vi "FTW-Actor.vi"(0 "FTW-TestExecutive-Core":refnum<class "FTW-TestExecutive-Core.lvclass">, 5 "FTW Actor Instance Configuration":string="{\n  \"Identity\": \"FTW Test Executive\",\n  \"InboxAddress\": \"inproc://ftwTestExec\",\n  \"LoggerAddress\": \"\",\n  \"Connections\": {},\n  \"Publishers\": {},\n  \"Subscriptions\": {},\n  \"Step Name Dictionary\": {},\n  \"Refresh Period\": 0.1\n}", 11 "ErrorIn":errorcluster) -> (15 "Error":errorcluster)   [LabVIEW 2015, in "FTW-TestExecutive-Core.lvclass"]
uses:
  FTW-TestExecutive-Core.lvclass
  FTW-TestExecutive-Results.ctl
  FTW-TestExecutive-Core.lvclass/FTW-TestExecutive-Core.ctl
  FTW-TestExecutive-Core_State.ctl
  FTW-TestExecutive-Step-State.ctl
  source/actor/Instance/FTW-ActorInstance.lvclass/FTW-ActorInstance.ctl
  source/JSON/core/FTW-JSON-Core-EncodingFlags.vi
  source/JSON/FTW-JSON-Parse.vi
  source/Reflection/FTW-Reflection-Type.vi
  source/CodeGen/JSON Deserialize/FTW-JSON-Core-GetFlattenedValue.vi
  source/actor/JobSequencer/FTW-SEQ-Current.vi
  source/CodeGen/JSON Deserialize/FTW-JSON-Deserialize.xnode
  source/actor/Message/Base/FTW-Message.lvclass
  source/actor/Connector/FTW-ActorConnector.lvclass
  source/actor/Instance/FTW-ActorInstance.lvclass
  source/actor/Message/Request/FTW-Message-IncomingRequest.lvclass
  source/actor/Instance-Extended/FTW-ActorExtended.lvclass
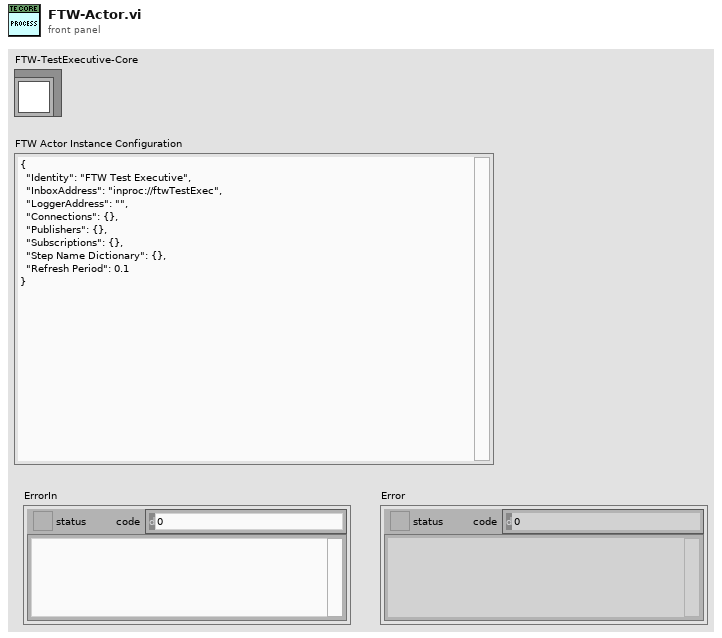
[diagram p1: front panel]
types:
  T1 = cluster{"Incoming Requests":refnum<event-registration>, "Local Messages":refnum<event-registration>, "Subscriber Registration":refnum<event-registration>}
  T2 = typedef "FTW-TestExecutive-Results.ctl" = cluster{"Start Time":timestamp, "Elapsed Time":dbl, "Passed":bool}
  T3 = typedef "FTW-TestExecutive-Step-State.ctl" = enum8{"None", "Failed", "Passed", "Timed out", "Aborted"}
  T4 = typedef "FTW-TestExecutive-Core.lvclass/FTW-TestExecutive-Core_State.ctl" = enum8{"Unloaded", "Loaded", "Executing", "Paused"}
  T5 = typedef "FTW-TestExecutive-Step.ctl" = cluster{"Name":string, "Type":string, "Config":string, "Elapsed Time":dbl, "Passed":bool, "State":T3, "Results":T2}
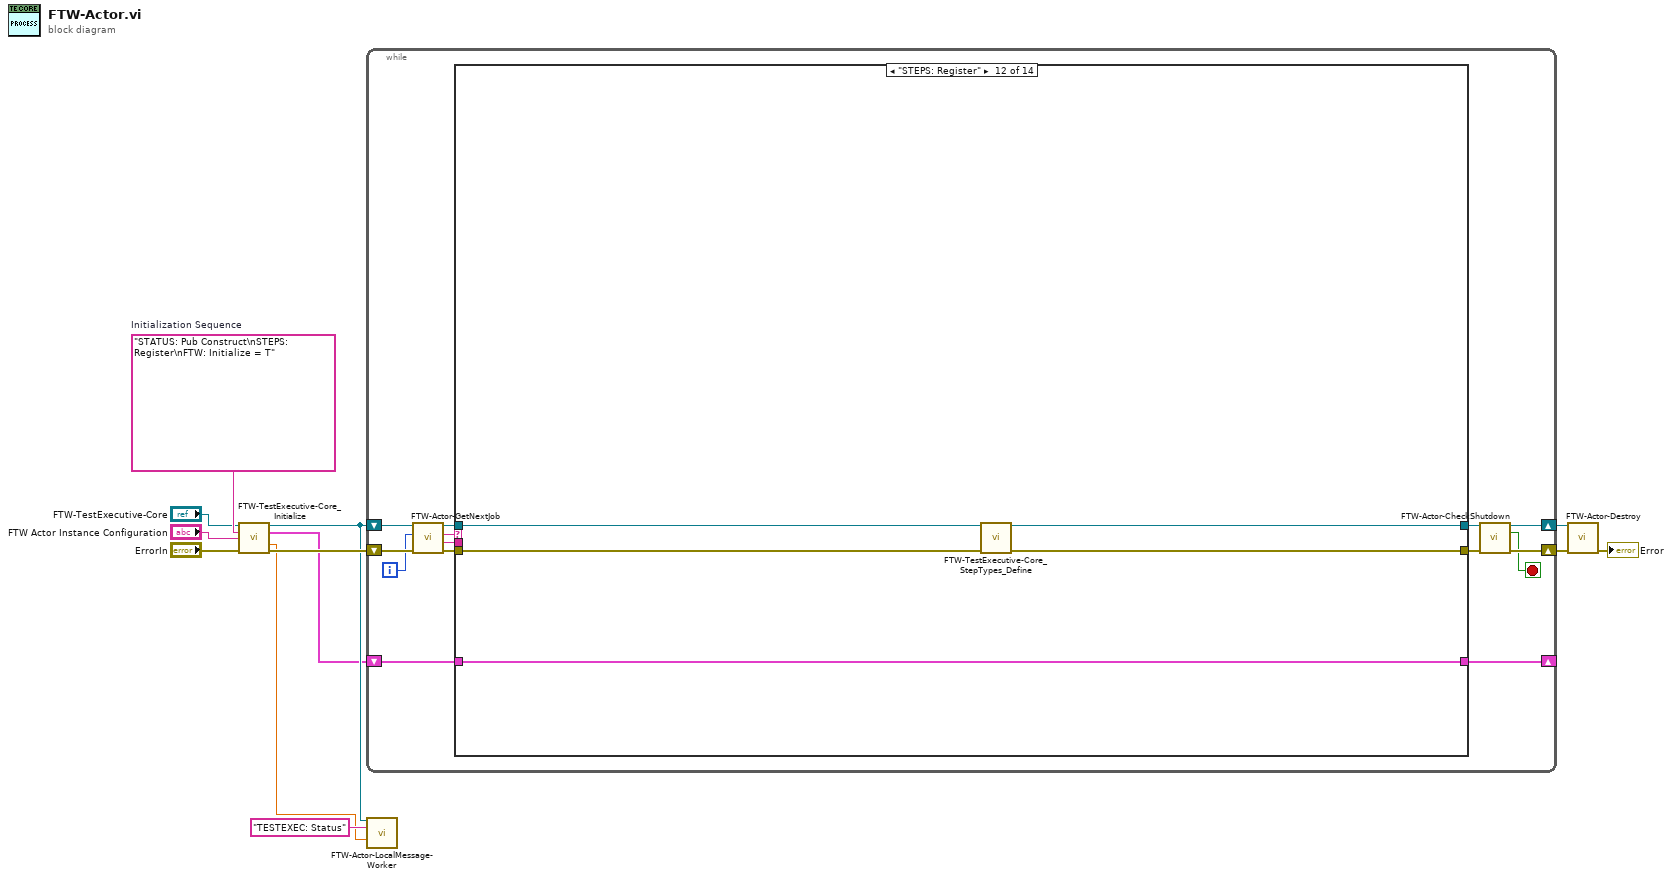
[diagram p0: block diagram]
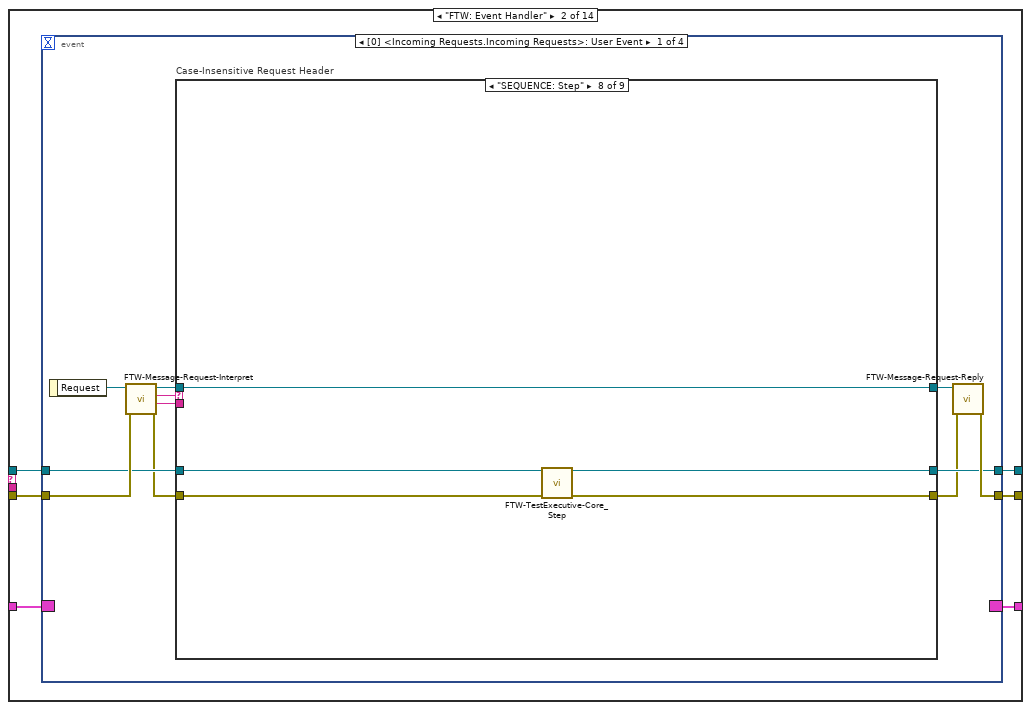
[diagram p3: hidden frame]
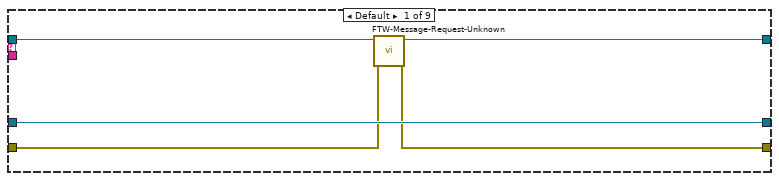
[diagram p4: hidden frame]
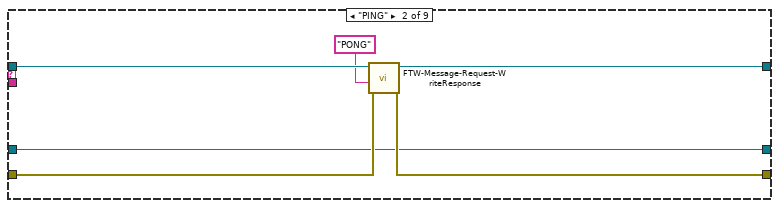
[diagram p5: hidden frame]
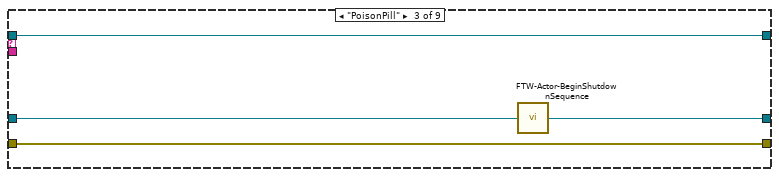
[diagram p6: hidden frame]
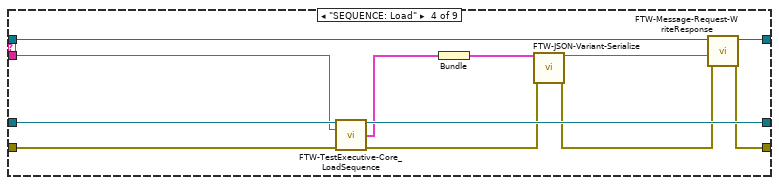
[diagram p7: hidden frame]
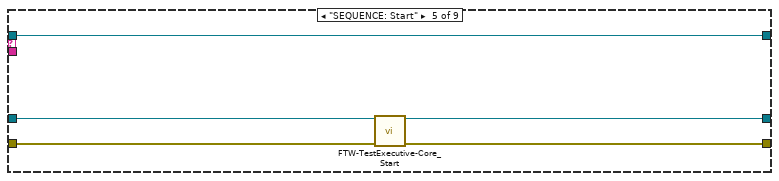
[diagram p8: hidden frame]
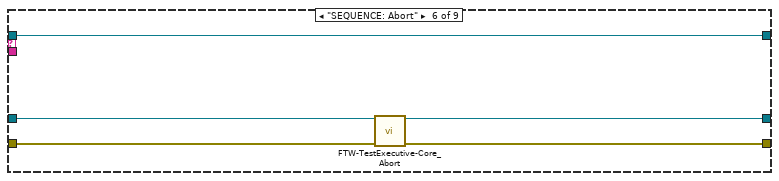
[diagram p9: hidden frame]
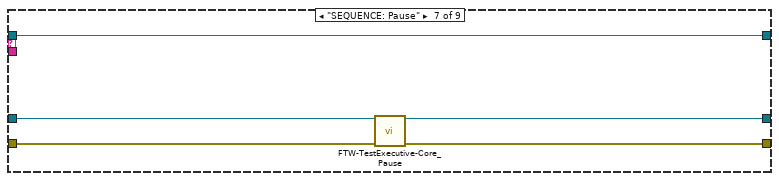
[diagram p10: hidden frame]
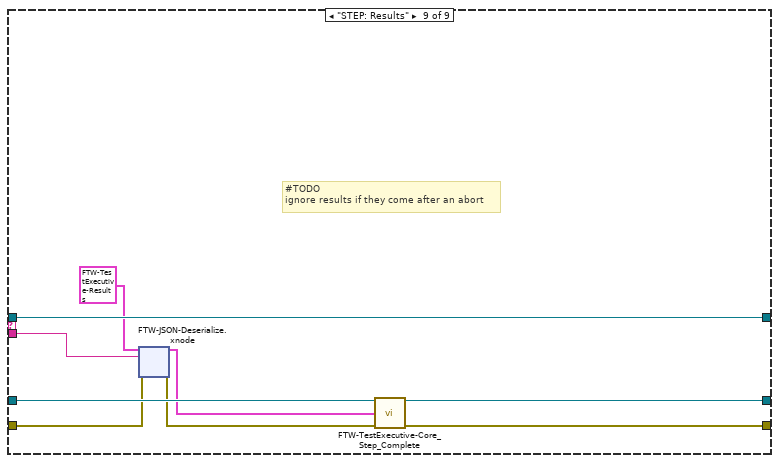
[diagram p11: hidden frame]
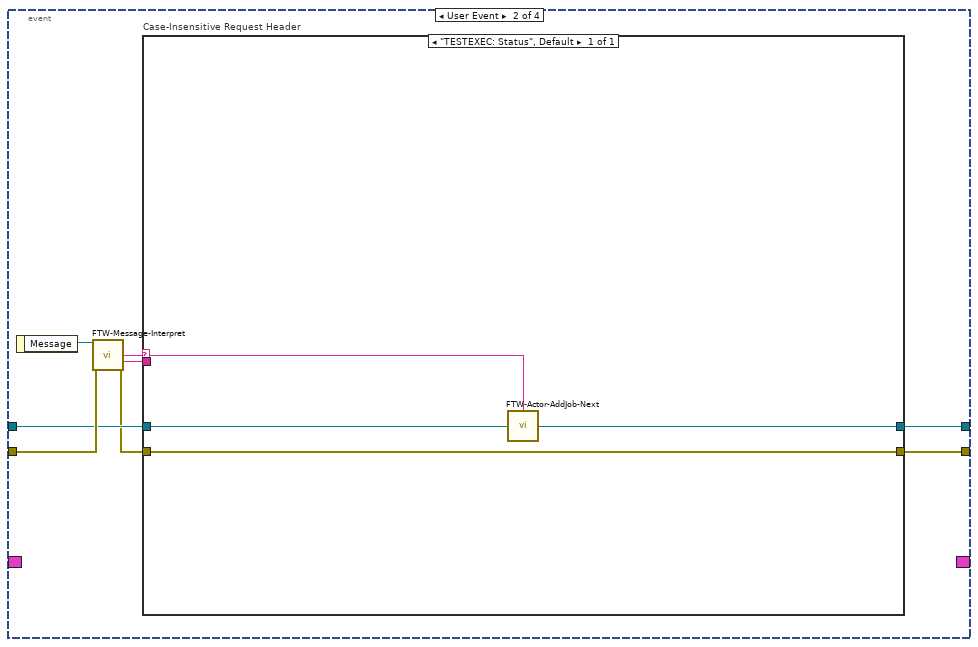
[diagram p12: hidden frame]
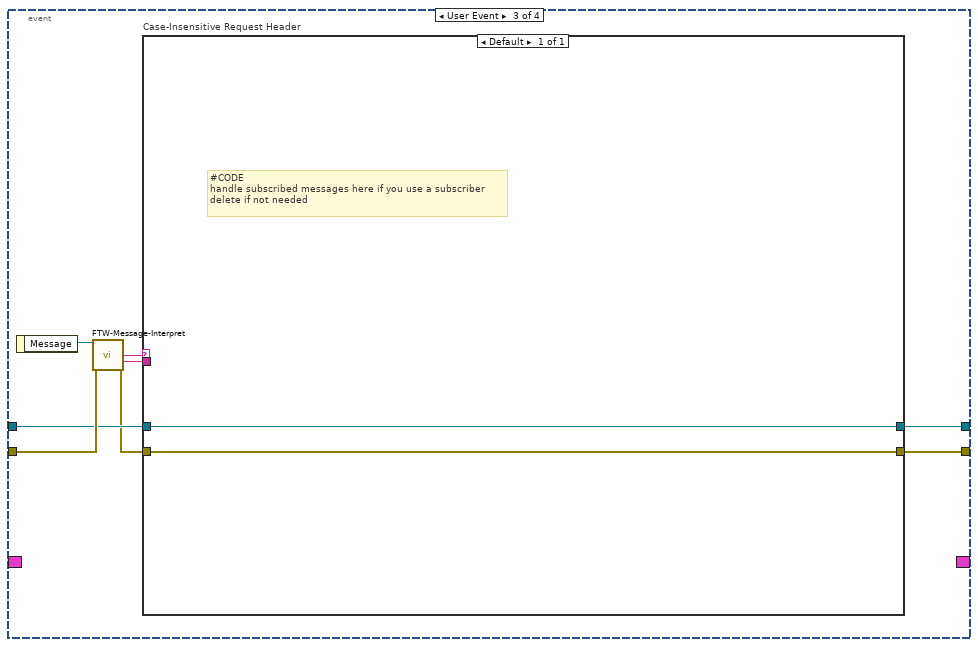
[diagram p13: hidden frame]
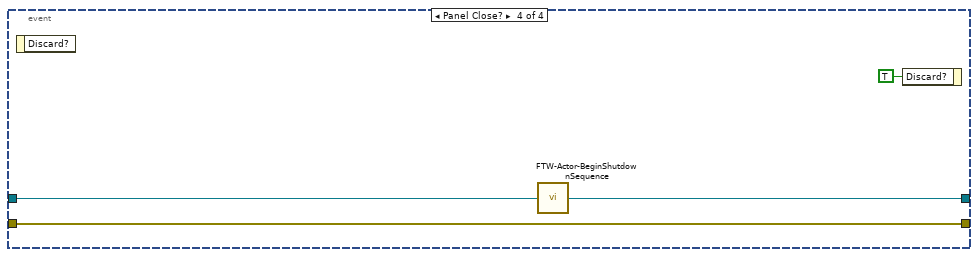
[diagram p14: hidden frame]
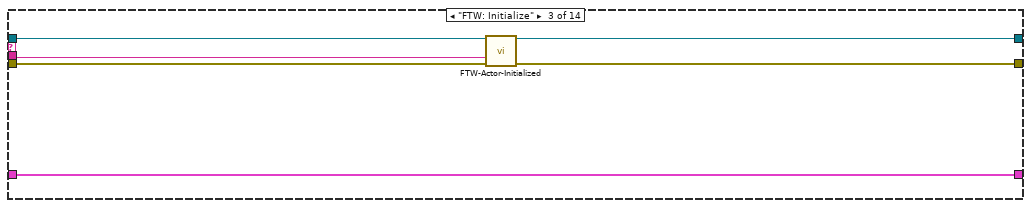
[diagram p15: hidden frame]
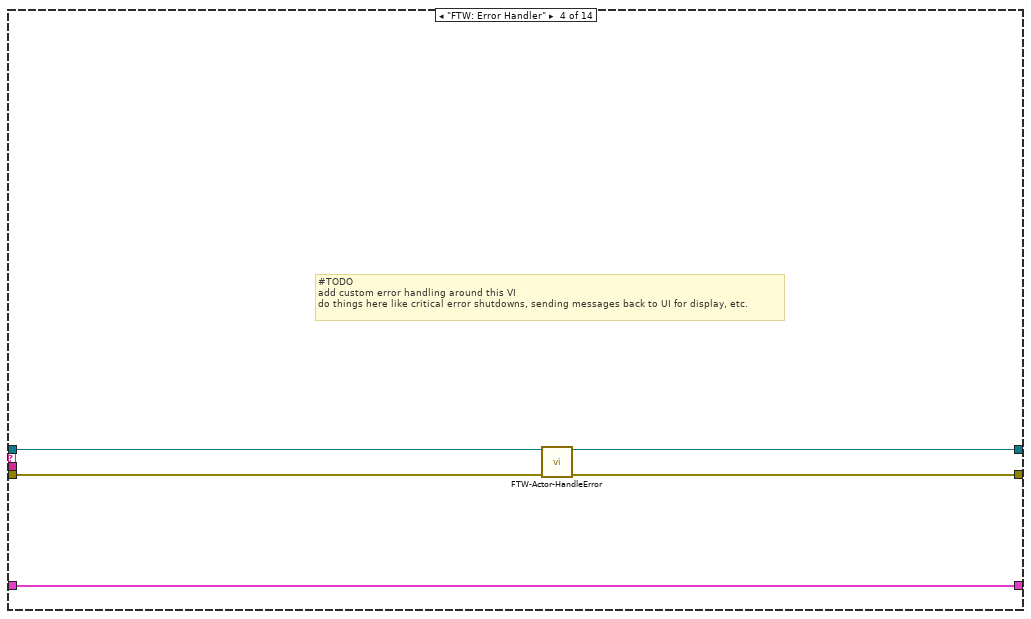
[diagram p16: hidden frame]
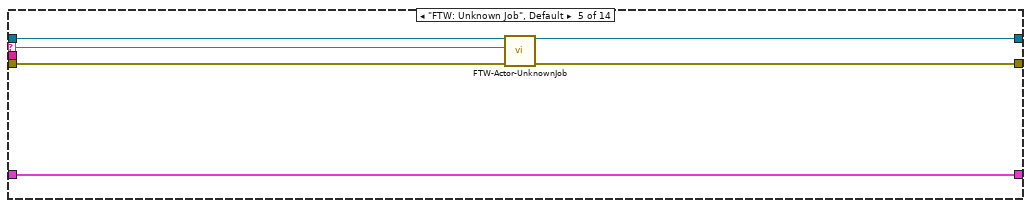
[diagram p17: hidden frame]
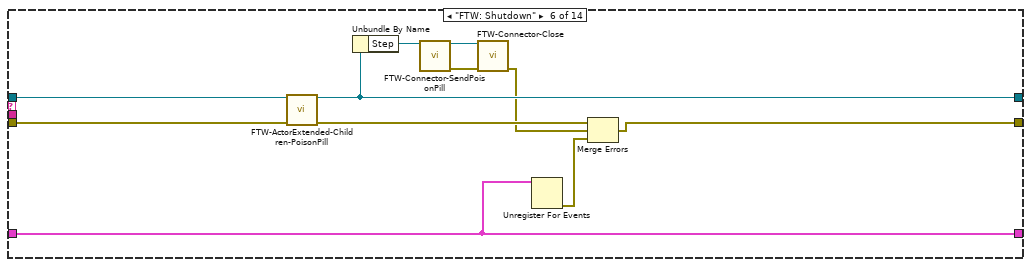
[diagram p18: hidden frame]
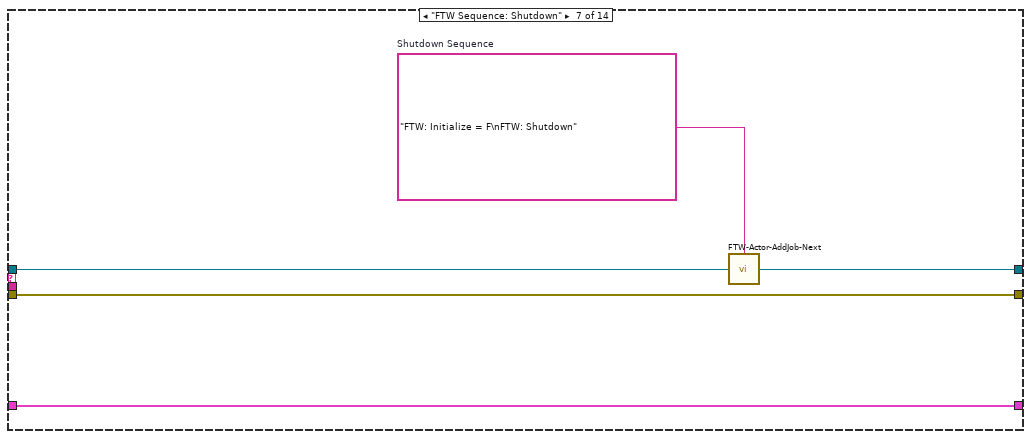
[diagram p19: hidden frame]
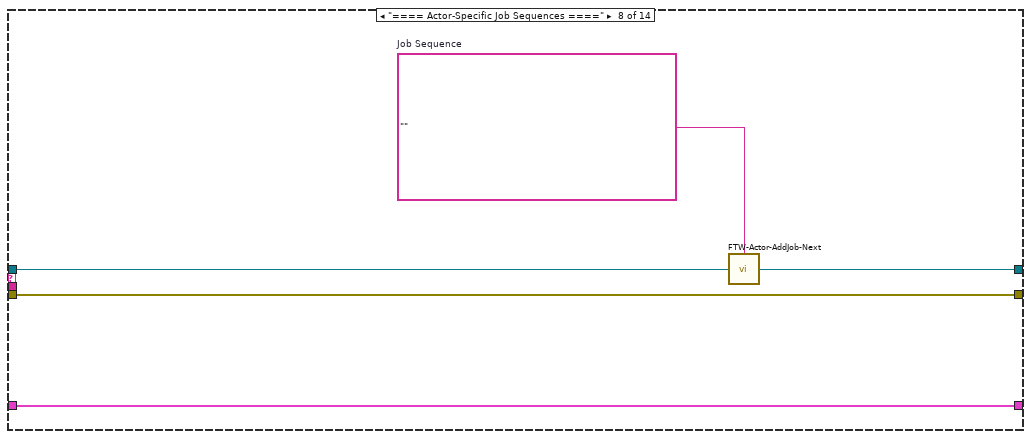
[diagram p20: hidden frame]
diagram:
  w2 = "STATUS: Pub Construct\nSTEPS: Register\nFTW: Initialize = T"  # Initialization Sequence
  n1 = call-dynamic "FTW-TestExecutive-Core_Initialize.vi"("Test Executive"="FTW-TestExecutive-Core", "Initialization Sequence"=w2, "FTW Actor Instance Configuration"="FTW Actor Instance Configuration", "error in (no error)"="ErrorIn") -> ("FTW-TestExecutive-Core Out"=w6:refnum<class "FTW-TestExecutive-Core.lvclass">, "Event Refnums"=w4:T1, "Refresh Period"=w5:dbl, "error out"=w9:errorcluster)  [unwired: 8 in]
  n2 = while {
    shift-right: [w16] -> w11
    shift-left: w9 -> [w23]
    shift-right: [w13] -> _
    shift-left: w4 -> [w26]
    shift-right: [w18] -> w12
    shift-left: w6 -> [w25]
    i -> [w14]
    stop <- w15 stop-if-true
    n3 = call "FTW-Actor-GetNextJob.vi"("error in"=w23, "Jobs Performed"=w14, "FTW Actor Instance"=w25) -> ("error out"=w22:errorcluster, "Job Data"=w20:string, "Job Name"=w21:string, "FTW Actor Instance out"=w24:refnum<class "FTW-TestExecutive-Core.lvclass">)  [unwired: 5 in]
    n4 = case shown="\"STEPS: Register\"" w21 {
      selector: w21 -> [_ _ _ _ w155 _ _ _ _ _ _ _ _ _]
      tunnel: [w28 w35 w146 w150 w158 w170 w175 w180 w184 w192 w222 w227 w232 w235] -> w17
      tunnel: w22 -> [w28 w34 w148 w152 w159 w171 w175 w180 w185 w191 w223 w228 w233 w241]
      tunnel: w26 -> [w29 w30 w149 w154 w160 w168 w176 w181 w186 w196 w224 w229 w234 w242]
      tunnel: [w29 w33 w149 w154 w160 w168 w176 w181 w186 w196 w224 w229 w234 w242] -> w13
      tunnel: w20 -> [_ _ w144 _ _ _ _ _ _ _ _ _ _ _]
      tunnel: [w27 w32 w147 w151 w156 w165 w173 w178 w182 w189 w221 w226 w231 w239] -> w19
      tunnel: w24 -> [w27 w31 w145 w153 w157 w166 w174 w179 w183 w190 w220 w225 w230 w240]
      frame "==== Featherweight Framework Jobs ====" {
      }
      frame "FTW: Event Handler" {
        n5 = event shown="[0] <Incoming Requests.Incoming Requests>: User Event" {
          selector: w30 -> [_ _ _ _]
          dyn-events: [_ _ _ _] -> w33
          timeout: _ -> [_ _ _ _]
          tunnel: [w45 w120 w132 w142] -> w35
          tunnel: w34 -> [w44 w124 w136 w142]
          tunnel: [w39 w121 w133 w140] -> w32
          tunnel: w31 -> [w43 w123 w135 w141]
          event User Event {
            n6 = event-data() -> ("Request"=w46:refnum<class "FTW-Message-IncomingRequest.lvclass">)  [unwired: 1 in]
            n7 = call "FTW-Message-Request-Interpret.vi"("error in"=w44, "FTW Incoming Request"=w46) -> ("error out"=w42:errorcluster, "Request Body"=w36:string, "Request Header"=w40:string, "FTW Incoming Request out"=w41:refnum<class "FTW-Message-IncomingRequest.lvclass">)  [unwired: 6 in]
            n8 = case "Case-Insensitive Request Header" shown="\"SEQUENCE: Step\"" w40 {
              tunnel: [w49 w55 w60 w64 w74 w79 w84 w89 w99] -> w38
              tunnel: w42 -> [w50 w56 w60 w70 w75 w80 w85 w90 w97]
              tunnel: [w51 w54 w61 w71 w76 w81 w86 w91 w100] -> w39
              tunnel: w43 -> [w51 w54 w59 w72 w77 w82 w87 w92 w101]
              tunnel: w41 -> [w48 w57 w58 w73 w78 w83 w88 w93 w102]
              tunnel: [w47 w53 w58 w68 w78 w83 w88 w93 w102] -> w37
              tunnel: w36 -> [_ _ _ w69 _ _ _ _ w98]
              frame Default {
                n9 = call "FTW-Message-Request-Unknown.vi"("error in"=w50, "FTW Incoming Request"=w48) -> ("error out"=w49:errorcluster, "FTW Incoming Request Out"=w47:refnum<class "FTW-Message-IncomingRequest.lvclass">)  [unwired: 8 in]
              }
              frame "PING" {
                n10 = call "FTW-Message-Request-WriteResponse.vi"("error in"=w56, "Response Body"="PONG" ("Response Header"), "FTW Incoming Request"=w57) -> ("error out"=w55:errorcluster, "FTW Incoming Request out"=w53:refnum<class "FTW-Message-IncomingRequest.lvclass">)  [unwired: 7 in]
              }
              frame "PoisonPill" {
                n11 = call "FTW-Actor-BeginShutdownSequence.vi"("FTW Actor Instance"=w59) -> ("FTW Actor Instance out"=w61:refnum<class "FTW-TestExecutive-Core.lvclass">)  [unwired: 3 in]
              }
              frame "SEQUENCE: Load" {
                n12 = call "FTW-TestExecutive-Core_LoadSequence.vi"("FTW-TestExecutive-Core In"=w72, "Sequence"=w69, "error in"=w70) -> ("FTW-TestExecutive-Core Out"=w71:refnum<class "FTW-TestExecutive-Core.lvclass">, "Loaded Sequence"=w62:T5[], "error out"=w67:errorcluster)  [unwired: 10 in]
                n13 = Bundle("Loaded Sequence"=w62) -> (w63:cluster{"Loaded Sequence":T5[]})  [unwired: 1 in]
                n14 = call "FTW-JSON-Variant-Serialize.vi"("Variant"=w63, "error in"=w67) -> ("JSON String"=w66:string, "error out"=w65:errorcluster)  [unwired: 12 in]
                n15 = call "FTW-Message-Request-WriteResponse.vi"("error in"=w65, "Response Body"=w66, "FTW Incoming Request"=w73) -> ("error out"=w64:errorcluster, "FTW Incoming Request out"=w68:refnum<class "FTW-Message-IncomingRequest.lvclass">)  [unwired: 7 in]
              }
              frame "SEQUENCE: Start" {
                n16 = call "FTW-TestExecutive-Core_Start.vi"("FTW-TestExecutive-Core In"=w77, "error in"=w75) -> ("FTW-TestExecutive-Core Out"=w76:refnum<class "FTW-TestExecutive-Core.lvclass">, "error out"=w74:errorcluster)  [unwired: 12 in]
              }
              frame "SEQUENCE: Abort" {
                n17 = call "FTW-TestExecutive-Core_Abort.vi"("FTW-TestExecutive-Core In"=w82, "error in"=w80) -> ("FTW-TestExecutive-Core Out"=w81:refnum<class "FTW-TestExecutive-Core.lvclass">, "error out"=w79:errorcluster)  [unwired: 12 in]
              }
              frame "SEQUENCE: Pause" {
                n18 = call "FTW-TestExecutive-Core_Pause.vi"("FTW-TestExecutive-Core In"=w87, "error in"=w85) -> ("FTW-TestExecutive-Core Out"=w86:refnum<class "FTW-TestExecutive-Core.lvclass">, "error out"=w84:errorcluster)  [unwired: 12 in]
              }
              frame "SEQUENCE: Step" {
                n19 = call "FTW-TestExecutive-Core_Step.vi"("FTW-TestExecutive-Core In"=w92, "error in"=w90) -> ("FTW-TestExecutive-Core Out"=w91:refnum<class "FTW-TestExecutive-Core.lvclass">, "error out"=w89:errorcluster)  [unwired: 12 in]
              }
              frame "STEP: Results" {
                # "#TODO\nignore results if they come after an abort"
                n20 = xnode "FTW-JSON-Deserialize.xnode"("Type and Defaults"=T2 {"Start Time"=timestamp(0 s since 1904-01-01), "Elapsed Time"=0.0, "Passed"=FALSE}, "JSON String"=w98, "error in"=w97) -> ("Values"=w95:T2, "error out"=w96:errorcluster)
                n21 = call "FTW-TestExecutive-Core_Step_Complete.vi"("FTW-TestExecutive-Core In"=w101, "Results"=w95, "error in"=w96) -> ("FTW-TestExecutive-Core Out"=w100:refnum<class "FTW-TestExecutive-Core.lvclass">, "error out"=w99:errorcluster)  [unwired: 11 in]
              }
            }
            n22 = call "FTW-Message-Request-Reply.vi"("FTW: Reply Error"=w38, "FTW Incoming Request"=w37) -> ("error out"=w45:errorcluster)  [unwired: 8 in, 1 out]
          }
          event User Event {
            n23 = event-data() -> ("Message"=w125:refnum<class "FTW-Message.lvclass">)  [unwired: 1 in]
            n24 = call-dynamic "FTW-Message-Interpret.vi"("FTW Message"=w125, "error in"=w124) -> ("Message Header"=w119:string, "Message Body"=w118:string, "error out"=w122:errorcluster)  [unwired: 9 in, 2 out]
            n25 = case "Case-Insensitive Request Header" shown="\"TESTEXEC: Status\", Default" w119 {
              selector: w119 -> [w126]
              tunnel: [w128] -> w120
              tunnel: w122 -> [w128]
              tunnel: [w127] -> w121
              tunnel: w123 -> [w129]
              tunnel: w118 -> [_]
              frame "TESTEXEC: Status", Default {
                n26 = call "FTW-Actor-AddJob-Next.vi"("Add Next in Job Queue"=w126, "FTW Actor Instance"=w129) -> ("FTW Actor Instance out"=w127:refnum<class "FTW-TestExecutive-Core.lvclass">)  [unwired: 2 in]
              }
            }
          }
          event User Event {
            n27 = event-data() -> ("Message"=w137:refnum<class "FTW-Message.lvclass">)  [unwired: 1 in]
            n28 = call-dynamic "FTW-Message-Interpret.vi"("FTW Message"=w137, "error in"=w136) -> ("Message Header"=w131:string, "Message Body"=w130:string, "error out"=w134:errorcluster)  [unwired: 9 in, 2 out]
            n29 = case "Case-Insensitive Request Header" shown="Default" w131 {
              tunnel: [w138] -> w132
              tunnel: w134 -> [w138]
              tunnel: [w139] -> w133
              tunnel: w135 -> [w139]
              tunnel: w130 -> [_]
              frame Default {
                # "#CODE\nhandle subscribed messages here if you use a subscriber\ndelete if not needed"
              }
            }
          }
          event Panel Close? {
            n30 = event-data() -> ()  [unwired: 1 in, 1 out]
            n31 = call "FTW-Actor-BeginShutdownSequence.vi"("FTW Actor Instance"=w141) -> ("FTW Actor Instance out"=w140:refnum<class "FTW-TestExecutive-Core.lvclass">)  [unwired: 3 in]
            n32 = event-data("Discard?"=TRUE) -> ()  [unwired: 1 in, 1 out]
          }
        }
      }
      frame "FTW: Initialize" {
        n33 = call-dynamic "FTW-Actor-Initialized.vi"("FTW Actor Instance"=w145, "Positive Init?"=w144, "error in"=w148) -> ("FTW Actor Instance out"=w147:refnum<class "FTW-TestExecutive-Core.lvclass">, "error out"=w146:errorcluster)  [unwired: 11 in]
      }
      frame "FTW: Error Handler" {
        # "#TODO\nadd custom error handling around this VI\ndo things here like critical error shutdowns, sending messages back to UI for display, etc."
        n34 = call-dynamic "FTW-Actor-HandleError.vi"("FTW Actor Instance"=w153, "error in"=w152) -> ("FTW Actor Instance out"=w151:refnum<class "FTW-TestExecutive-Core.lvclass">, "error out"=w150:errorcluster)  [unwired: 10 in, 2 out]
      }
      frame "FTW: Unknown Job", Default {
        n35 = call-dynamic "FTW-Actor-UnknownJob.vi"("FTW Actor Instance"=w157, "Unknown Job"=w155, "error in"=w159) -> ("FTW Actor Instance out"=w156:refnum<class "FTW-TestExecutive-Core.lvclass">, "error out"=w158:errorcluster)  [unwired: 11 in]
      }
      frame "FTW: Shutdown" {
        n36 = call "FTW-ActorExtended-Children-PoisonPill.vi"("FTW-ActorExtended In"=w166, "error in"=w171) -> ("FTW-ActorExtended Out"=w165:refnum<class "FTW-TestExecutive-Core.lvclass">, "error out"=w167:errorcluster)  [unwired: 12 in]
        n37 = Unbundle By Name(w165) -> ("Step"=w164:refnum<class "FTW-ActorConnector.lvclass">)
        n38 = call-dynamic "FTW-Connector-SendPoisonPill.vi"("FTW Actor Connector"=w164) -> ("FTW Actor Connector out"=w163:refnum<class "FTW-ActorConnector.lvclass">, "error out"=w162:errorcluster)  [unwired: 9 in, 4 out]
        n39 = call-dynamic "FTW-Connector-Close.vi"("FTW Actor Connector"=w163, "error in"=w162) -> ("error out"=w161:errorcluster)  [unwired: 13 in]
        n40 = Unregister For Events(event registration refnum=w168) -> (error out=w169:errorcluster)  [unwired: 1 in]
        n41 = Merge Errors(w167, w161, w169) -> (w170:errorcluster)
      }
      frame "FTW Sequence: Shutdown" {
        w172 = "FTW: Initialize = F\nFTW: Shutdown"  # Shutdown Sequence
        n42 = call "FTW-Actor-AddJob-Next.vi"("Add Next in Job Queue"=w172, "FTW Actor Instance"=w174) -> ("FTW Actor Instance out"=w173:refnum<class "FTW-TestExecutive-Core.lvclass">)  [unwired: 2 in]
      }
      frame "==== Actor-Specific Job Sequences ====" {
        w177 = ""  # Job Sequence
        n43 = call "FTW-Actor-AddJob-Next.vi"("Add Next in Job Queue"=w177, "FTW Actor Instance"=w179) -> ("FTW Actor Instance out"=w178:refnum<class "FTW-TestExecutive-Core.lvclass">)  [unwired: 2 in]
      }
      frame "==== Actor-Specific Jobs ====" {
        # "use this job as the template for other jobs"
        n44 = in-place {
          n45 = in-place-cluster #1(w183) -> ("State"=w187:T4)
          n46 = in-place-match #2(w185) -> (w188:errorcluster)
          n47 = in-place-cluster #1("State"=w187) -> (w182:refnum<class "FTW-TestExecutive-Core.lvclass">)
          n48 = in-place-match #2(w188) -> (w184:errorcluster)
        }
      }
      frame "TESTEXEC: Status" {
        n49 = Unbundle By Name(w190) -> ("State"=w194:T4, "Step Start Time"=w195:dbl, "Step Timeout"=w193:dbl)
        n50 = case shown="\"Executing\"" w194 {
          tunnel: w195 -> [_ w206 _]
          tunnel: w193 -> [_ w204 _]
          tunnel: [w197 w201 w216] -> w192
          tunnel: w191 -> [w197 w203 w216]
          tunnel: w190 -> [w198 w200 w217]
          tunnel: [w198 w202 w217] -> w189
          frame "Unloaded", "Loaded" {
          }
          frame "Executing" {
            n51 = call "FTW-Time-Uptime.vi"("Previous Uptime"=w206) -> ("Elapsed Time"=w205:dbl)  [unwired: 12 in, 2 out]
            n52 = Greater?(x=w205, y=w204) -> (0:w199:bool)
            n53 = case shown="True" w199 {
              tunnel: w203 -> [w207 w215]
              tunnel: [w208 w214] -> w202
              tunnel: [w207 w212] -> w201
              tunnel: w200 -> [w208 w211]
              frame False {
              }
              frame True {
                n54 = call "FTW-TestExecutive-Core_Step_SetStatus.vi"("FTW-TestExecutive-Core In"=w211, "State"=FTW-TestExecutive-Step-State."Timed out", "error in"=w215) -> ("FTW-TestExecutive-Core Out"=w210:refnum<class "FTW-TestExecutive-Core.lvclass">, "error out"=w212:errorcluster)  [unwired: 11 in]
                n55 = Bundle By Name(cluster=w210, "State"=FTW-TestExecutive-Core_State."Loaded") -> (w214:refnum<class "FTW-TestExecutive-Core.lvclass">)
              }
            }
          }
          frame "Paused" {
          }
        }
      }
      frame "STATUS: Pub Construct" {
        # "add status publisher for test exec"
        n56 = call "FTW-ActorExtended-Publisher-Add.vi"("FTW-ActorExtended In"=w220, "Publisher Name"="TestExecStatusPub", "Publisher URI"="inproc://*", "error in"=w223) -> ("FTW-ActorExtended Out"=w221:refnum<class "FTW-TestExecutive-Core.lvclass">, "error out"=w222:errorcluster)  [unwired: 10 in]
      }
      frame "STEPS: Register" {
        n57 = call-dynamic "FTW-TestExecutive-Core_StepTypes_Define.vi"("FTW-TestExecutive-Core In"=w225, "error in"=w228) -> ("FTW-TestExecutive-Core Out"=w226:refnum<class "FTW-TestExecutive-Core.lvclass">, "error out"=w227:errorcluster)  [unwired: 12 in]
      }
      frame "STEP: Execute" {
        n58 = call "FTW-TestExecutive-Core_Step_Launch.vi"("FTW-TestExecutive-Core In"=w230, "error in"=w233) -> ("FTW-TestExecutive-Core Out"=w231:refnum<class "FTW-TestExecutive-Core.lvclass">, "error out"=w232:errorcluster)  [unwired: 12 in]
      }
      frame "CONN: Ask" {
        # "example of asking a connected actor something\n\nuse the connection to call the actor API"
        n59 = call "FTW-ActorExtended-Connection-Get.vi"("FTW-ActorExtended In"=w240, "Connector Name"="ConnectionOne" ("Publisher Name"), "error in"=w241) -> ("FTW-ActorExtended Out"=w239:refnum<class "FTW-TestExecutive-Core.lvclass">, "FTW Actor Connector"=w237:refnum<class "FTW-ActorConnector.lvclass">, "error out"=w236:errorcluster)  [unwired: 10 in]
        n60 = flat-sequence {
          tunnel: w237 -> [_]
          tunnel: w236 -> [w243]
          tunnel: [w243] -> w235
          frame #0 {
          }
        }
      }
    }
    n61 = call "FTW-Actor-CheckShutdown.vi"("FTW Actor Instance"=w19, "error in"=w17) -> ("FTW Actor Instance out"=w18:refnum<class "FTW-TestExecutive-Core.lvclass">, "Shutdown?"=w15:bool, "error out"=w16:errorcluster)  [unwired: 11 in]
  }
  n62 = call-dynamic "FTW-Actor-LocalMessage-Worker.vi"("FTW-ActorInstance In"=w6, "Message Header"="TESTEXEC: Status", "Send Rate"=w5) -> ()  [unwired: 13 in]
  n63 = call-dynamic "FTW-Actor-Destroy.vi"("FTW Actor Instance"=w12, "error in"=w11) -> ("error out"=→"Error":errorcluster)  [unwired: 13 in]
